vi "CalcCC.vi"(6 "Signal Fraction":dbl, 8 "session in":refnum<k35>, 9 "Specimem":enum16{"Please Select Value", "NH3", "ND3"}(ring), 10 "Input Signal":dbl[][](array[numeric]), 11 "Take CC":bool) -> (0 "session out":refnum<k35>)   [LabVIEW 2018]
panel:
  in  "Script Path":path=path "C:/Users/Ptgroup/Documents/UVA-Lab-Software/LANL-System/rssmt/Python_Files/db.py"
  out "Error Message":string
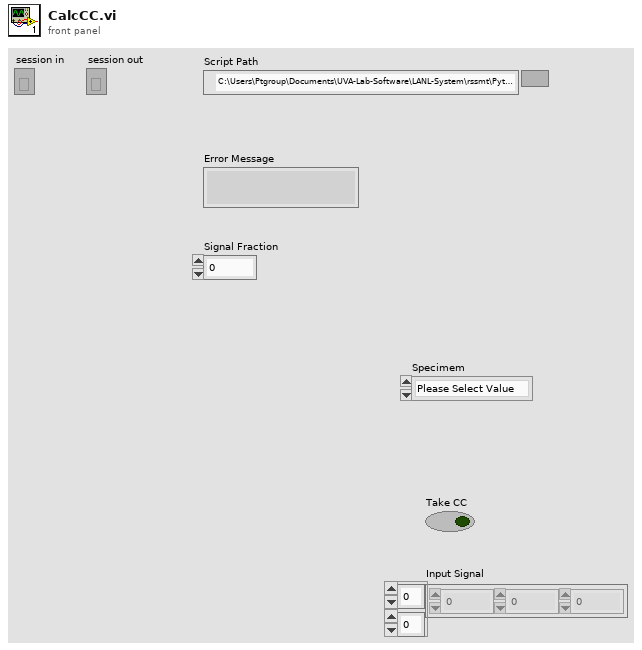
[diagram p1: front panel]
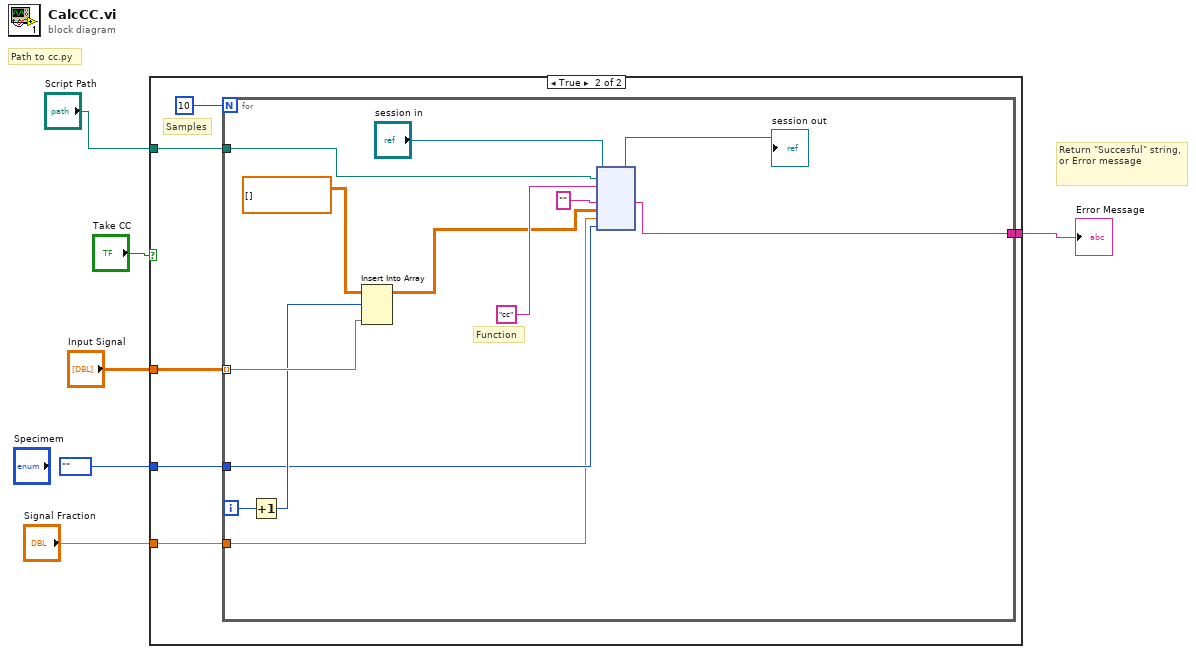
[diagram p0: block diagram]
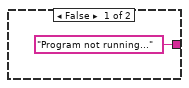
[diagram p2: hidden frame]
diagram:
  # "Return \"Succesful\" string, or Error message"
  # "Path to cc.py"
  n1 = case shown="True" "Take CC" {
    tunnel: "Input Signal" -> [_ w12]
    tunnel: "Script Path" -> [_ w11]
    tunnel: ["Program not running..." w10] -> w3
    tunnel: enum16{""}."" -> [_ w9]
    tunnel: "Signal Fraction" -> [_ w8]
    frame False {
    }
    frame True {
      # "Samples"
      n2 = for {
        N: 10 -> [_]
        tunnel: w12 -> [w25] mode=indexing
        tunnel: w11 -> [w19]
        tunnel: [w18] -> w10
        tunnel: w9 -> [w15]
        tunnel: w8 -> [w14]
        i -> [w24]
        # "Function"
        n3 = Increment(x=w24) -> (x+1=w23:i32)
        n4 = Insert Into Array(array=dbl[][] [] ("Signals"), index (row)=w23, new element=w25) -> (w16:dbl[][])  [unwired: 1 in]
        n5 = node("session in", w19, "cc" ("function name"), "", w16, w14, w15) -> (→"session out":refnum<k35>, w18:string)  [unwired: 4 in, 3 out]
      }
    }
  }
  "Error Message" <- w3
